vi "acquire double cursor window data.vi"(9 "z in":cdb[](array[numeric]), 10 "omega in":dbl[](array[numeric]), 11 "cursor window":T1={"left"=2378.60310421286, "right "=2421.6740576496672, "center"=2421.6740576496672, "window"=2421.6740576496672, "cursors"=[], "relative"=0, "absolute"=0, "fixed vertical offset"=2421.6740576496672, "vertical offset"=2421.6740576496672, "skew"=2421.6740576496672, "default window frac"=2421.6740576496672, "kind"=enum."fancy", "skew.left"=2421.6740576496672, "skew.right"=0.0, "Plot ref"=refnum, "wing order"=enum."back"}) -> (1 "z out":cdb[](array[numeric]), 2 "omega  out":dbl[](array[numeric]))   [LabVIEW 2010]
uses:
  cursor winow.ctl
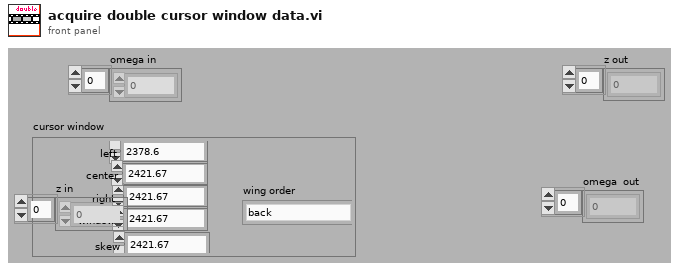
[diagram p1: front panel]
types:
  T1 = typedef "cursor winow.ctl" = cluster{"left":dbl, "right ":dbl, "center":dbl, "window":dbl, "cursors":i32[], "relative":i32, "absolute":i32, "fixed vertical offset":dbl, "vertical offset":dbl, "skew":dbl, "default window frac":dbl, "kind":enum16{"symmetric", "skewed", "fancy"}, "skew.left":dbl, "skew.right":dbl, "Plot ref":refnum<vi>, "wing order":enum16{"forw", "back"}}
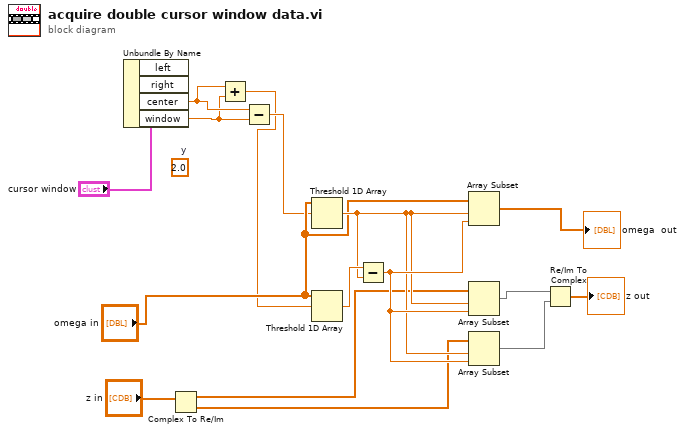
[diagram p0: block diagram]
diagram:
  (unwired) 2.0  # y
  n1 = Unbundle By Name("cursor window") -> ("center"=w4:dbl, "window"=w3:dbl)  [unwired: 2 out]
  n2 = Complex To Re/Im(x + iy="z in") -> (x=w9:dbl[], y=w8:dbl[])
  n3 = Add(x=w4, y=w3) -> (x+y=w1:dbl)
  n4 = Subtract(x=w4, y=w3) -> (x-y=w2:dbl)
  n5 = Threshold 1D Array(2:w2, 3:"omega in") -> (0:w14:dbl)  [unwired: 1 in]
  n6 = Threshold 1D Array(2:w1, 3:"omega in") -> (0:w16:dbl)  [unwired: 1 in]
  n7 = Subtract(x=w16, y=w14) -> (x-y=w15:dbl)
  n8 = Array Subset(array="omega in", index=w14, length=w15) -> (→"omega  out":dbl[])
  n9 = Array Subset(array=w9, index=w14, length=w15) -> (w12:dbl[])
  n10 = Array Subset(array=w8, index=w14, length=w15) -> (w13:dbl[])
  n11 = Re/Im To Complex(1:w13, 2:w12) -> (0:→"z out":cdb[])
